vi "Get VI Indivisual Error Code Table.vi"() -> (1 "Driver VI Individual Error Code Table":u16[][](array[numeric])=[[9999, 9999, 9999, 9999, 9999], [9999, 9999, 9999, 9999, 9999], [9999, 9999, 9999, 6700, 9999], [9999, 9999, 9999, 9999, 9999], [9999, 9999, 9999, 9999, 9999], [9999, 9999, 9999, 9999, 9999], [6500, 9999, 9999, 9999, 9999], [6501, 9999, 9999, 6701, 9999], [6501, 9999, 9999, 6701, 9999], [6503, 9999, 9999, 9999, 9999], [6503, 9999, 9999, 9999, 9999], [6503, 9999, 9999, 9999, 9999], [9999, 9999, 9999, 9999, 9999], [9999, 9999, 9999, 9999, 9999], [9999, 9999, 9999, 9999, 9999], [9999, 9999, 9999, 9999, 9999], [9999, 9999, 9999, 9999, 9999], [9999, 9999, 9999, 9999, 9999], [9999, 9999, 9999, 9999, 9999], [9999, 9999, 9999, 9999, 9999], [9999, 9999, 9999, 9999, 9999], [6502, 9999, 9999, 9999, 9999], [9999, 9999, 9999, 9999, 9999], [6503, 9999, 9999, 9999, 9999], [6504, 6505, 9999, 6702, 9999], [6504, 6506, 9999, 6703, 9999], [6503, 6505, 9999, 6702, 9999], [6503, 6506, 9999, 6703, 9999], [6503, 6507, 6508, 9999, 9999], [6503, 6507, 6508, 9999, 9999], [6503, 9999, 9999, 9999, 9999], [6503, 6509, 9999, 9999, 9999], [6503, 6510, 9999, 9999, 9999], [6503, 6511, 9999, 6704, 9999], [6504, 6512, 9999, 6705, 6706], [9999, 9999, 9999, 9999, 9999], [9999, 9999, 9999, 9999, 9999]])   [LabVIEW 2014, in "Keyence LJ-V7000.lvlib"]
uses:
  Keyence LJ-V7000.lvlib
panel:
  # "Initialize\nClose\nReboot Controller\nReturn to Factory State\nGet System Error\nClear System Error\nTrigger\nStart Batch Measurements\nStop Batch Measurements\nAuto Zero\nTiming\nReset\nClear Memory\nSet Setting\nGet Setting\nInitialize Setting\nReflect Setting\nUpdate Write Settings Area\nCheck Status of Saving to Save Area\nSet Time\nGet Time\nChange Program\nRead Active Program Number\nRead Measurement Data\nRead Profiles(for High-Speed Mode)\nRead Batch Profiles(for High-Speed Mode)\nRead Profiles(for Advanced Mode)\nRead Batch Profiles(for Advanced Mode)\nStart Storage\nStop Storage\nRead Storage Status\nRead Data Storage Data\nRead Profile Storage Data\nRead Batch Profile Storage Data\nStart High-Speed Data Communication\nStop High-Speed Data Communication\nRead Profiles(for High-Speed Communication)"
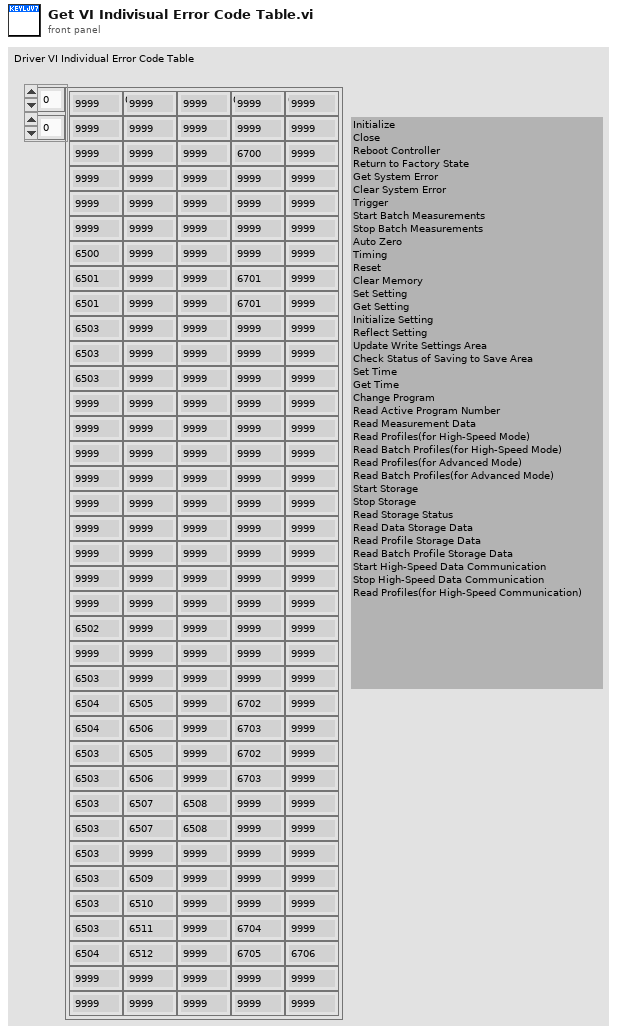
[diagram p1: front panel]
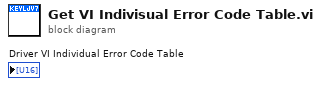
[diagram p0: block diagram]
diagram:
